vi "Panel Output Voltage Test.vi"(8 "Error In":errorcluster, 10 "Channel":i32=6, 11 "DMM In":string="DMM") -> (0 "Error Out":errorcluster, 3 "Voltage":dbl)   [LabVIEW 2015]
uses:
  <instrlib>/Driver Simulation/DMM/Signal Types.ctl
  <instrlib>/Driver Simulation/DMM.lvlib
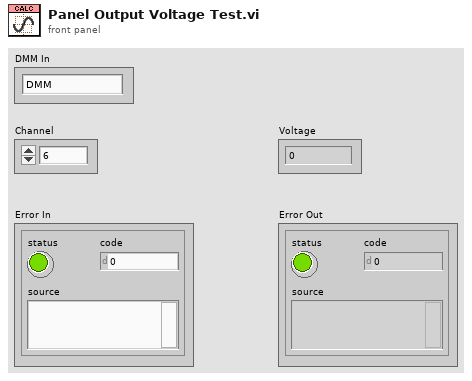
[diagram p1: front panel]
types:
  T1 = typedef "Driver Simulation.lvlib/DMM.lvlib/Signal Types.ctl" = enum16{"DC", "AC"}
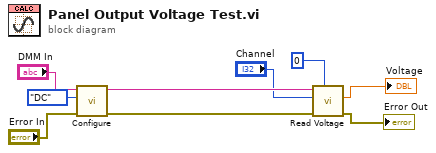
[diagram p0: block diagram]
diagram:
  n1 = call <instrlib>:"Configure.vi"("error in (no error)"="Error In", "Signal Type"=Signal_Types."DC", "DMM in"="DMM In") -> ("error out"=w8:errorcluster, "DMM out"=w9:string)  [unwired: 7 in]
  n2 = call <instrlib>:"Read Voltage.vi"("Test Socket (0)"=0, "error in (no error)"=w8, "Channel"="Channel", "DMM in"=w9) -> ("error out"=→"Error Out":errorcluster, "Voltage"=→"Voltage":dbl)  [unwired: 5 in, 1 out]
